vi "JGPR2.vi"() -> ()   [LabVIEW 2019]
doc: "This VI allows you to load data and graph it by raw data then gives you the fft graph and also allows for diffrent types of windowing of the data you can also look at data in frequency domain and save the data"
uses:
  <vilib>/Analysis/NI_AALPro.lvlib
panel:
  out "rate (Hz)":dbl format="%#_3g"
  in  "Window type":enum16{"Hanning", "Hamming", "Blackman"}(ring)
  out "interval (s)":dbl format="%#_3g"
  in  "Lin/dB":bool caption="Power spectrun presentation"
  in  "Tabs":T1(tab)
  out "Raw Data Graph":cluster{dbl, dbl, dbl[]}(graph)
  out "Data to FFT":cluster{dbl, dbl, "Windowed X":dbl[]}(graph)
  out "Power Spectrum":cluster{dbl, "df":dbl, "data out":dbl[]}(graph)
  out "data to save":dbl[][](array[numeric]) format="%#_3e"
  in  "Comments for header":string="This data is ....."
  in  "Windowing":bool
  out "raw data":dbl[][](array[numeric])
  out "Raw Data File Header":string
  in  "exit without save":bool
  in  "exit early":bool
  in  "save data":bool
  in  "load raw data":bool
  # "Post-processing of Data"
  # "Source data"
  # "File Output"
  # "raw"
  # "into PS"
  # "out of PS"
  # "Juan Gamez\nP3600\nCSUSB Physics"
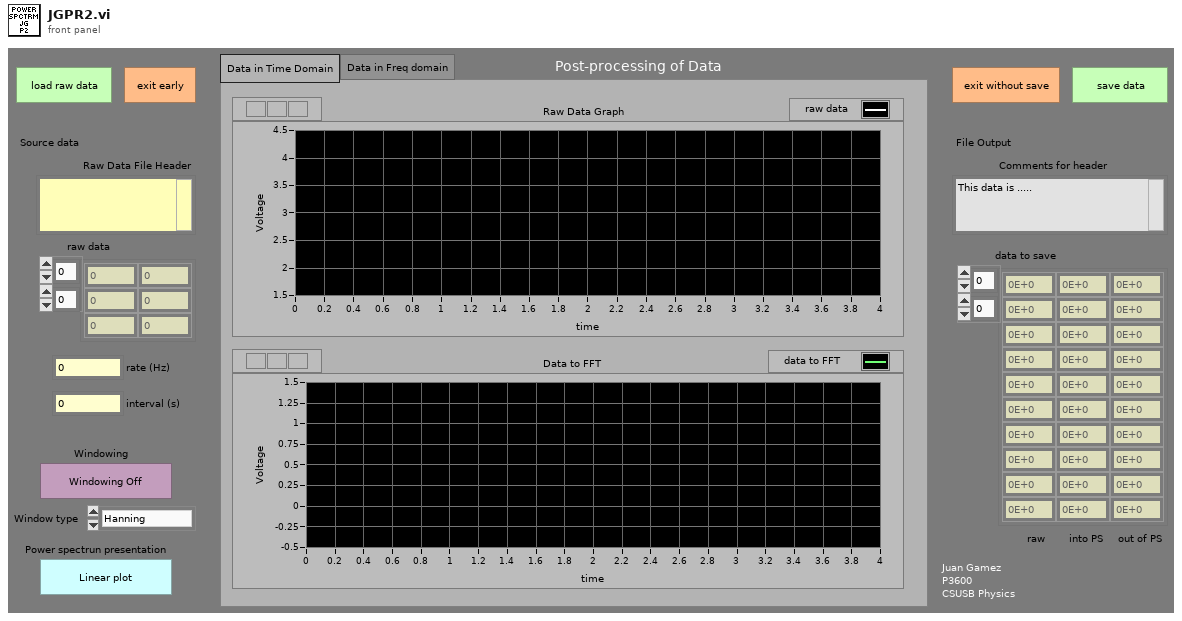
[diagram p1: front panel]
types:
  T1 = enum32{"Data in Time Domain", "Data in Freq domain"}
  T2 = cluster{dbl, "Interval (s)":dbl, "windowed data out":dbl[]}
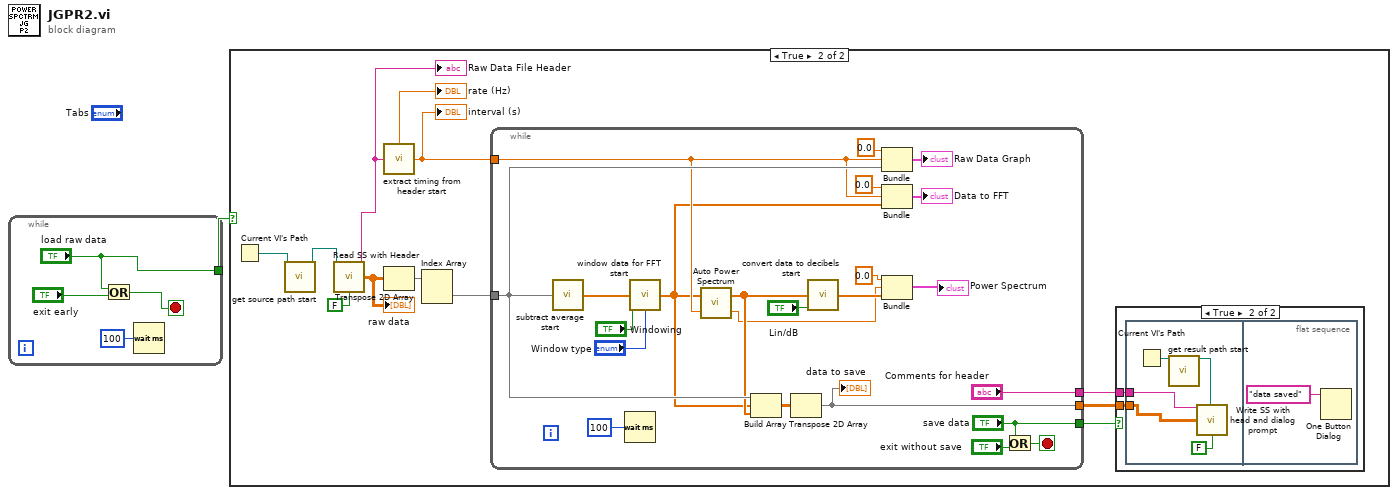
[diagram p0: block diagram]
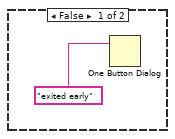
[diagram p2: hidden frame]
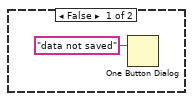
[diagram p3: hidden frame]
diagram:
  n1 = while {
    tunnel: ["load raw data"] -> w1
    stop <- w3 stop-if-true
    n2 = Or(x="load raw data", y="exit early") -> (x .or. y?=w3:bool)
    n3 = Wait (ms)(milliseconds to wait=u32 100) -> ()  [unwired: 1 out]
  }
  n4 = case shown="True" w1 {
    frame False {
      n5 = One Button Dialog(message="exited early") -> ()  [unwired: 1 in, 1 out]
    }
    frame True {
      n6 = Current VI's Path() -> (path=w11:path)
      n7 = call "get source path start.vi"("main VI path"=w11) -> ("source file path"=w10:path)  [unwired: 14 in]
      n8 = call "Read SS with Header.vi"("file path"=w10, "use int dialog (default=T)"=FALSE) -> ("Header String"=w14:string, "Data Read"=w18:dbl[][])  [unwired: 11 in, 1 out]
      "raw data" <- w18
      "Raw Data File Header" <- w14
      n9 = call "extract timing from header start.vi"("Header String"=w14) -> ("Rate (Hz)"=→"rate (Hz)":dbl, "Interval (s)"=w13:dbl)  [unwired: 13 in]
      "interval (s)" <- w13
      n10 = Transpose 2D Array(2D array=w18) -> (transposed array=w17:dbl[][])
      n11 = Index Array(array=w17) -> (element=w16:dbl[])  [unwired: 2 in]
      n12 = while {
        tunnel: w16 -> [w41]
        tunnel: ["save data"] -> w9
        tunnel: [w46] -> w7
        tunnel: ["Comments for header"] -> w8
        tunnel: w13 -> [w36]
        stop <- w48 stop-if-true
        n13 = call "subtract average start.vi"("data in"=w41) -> ("data with zero average out"=w35:dbl[])  [unwired: 14 in]
        n14 = Wait (ms)(milliseconds to wait=u32 100) -> ()  [unwired: 1 out]
        n15 = call "window data for FFT start.vi"("data in"=w35, "Windowing ON"="Windowing", "Window type"="Window type") -> ("windowed data out"=w34:dbl[])  [unwired: 12 in]
        n16 = call <vilib>:"Auto Power Spectrum.vi"("dt"=w36, "Signal (V)"=w34) -> ("df"=w29:dbl, "Power Spectrum (V^2 rms)"=w40:dbl[])
        n17 = Build Array(w41, w34, w40) -> (w39:dbl[][])
        n18 = Transpose 2D Array(2D array=w39) -> (transposed array=w46:dbl[][])
        "data to save" <- w46
        n19 = call "convert data to decibels start.vi"("data in"=w40, "Lin/dB"="Lin/dB") -> ("data out"=w30:dbl[])  [unwired: 13 in]
        n20 = Bundle(0.0, "Interval (s)"=w36, w41) -> (→"Raw Data Graph":cluster{dbl, "Interval (s)":dbl, dbl[]})  [unwired: 1 in]
        n21 = Bundle(0.0, "Interval (s)"=w36, "windowed data out"=w34) -> (→"Data to FFT":T2)  [unwired: 1 in]
        n22 = Bundle(0.0, "df"=w29, "data out"=w30) -> (→"Power Spectrum":cluster{dbl, "df":dbl, "data out":dbl[]})  [unwired: 1 in]
        n23 = Or(x="save data", y="exit without save") -> (x .or. y?=w48:bool)
      }
      n24 = case shown="True" w9 {
        tunnel: w8 -> [_ w21]
        tunnel: w7 -> [_ w20]
        frame False {
          n25 = One Button Dialog(message="data not saved") -> ()  [unwired: 1 in, 1 out]
        }
        frame True {
          n26 = flat-sequence {
            tunnel: w21 -> [w23]
            tunnel: w20 -> [w22]
            frame #0 {
              n27 = Current VI's Path() -> (path=w26:path)
              n28 = call "get result path start.vi"("main VI path"=w26) -> ("result file path"=w24:path)  [unwired: 14 in]
              n29 = call "Write SS with head and dialog prompt.vi"("Header String"=w23, "file path"=w24, "Data to Write"=w22, "use int dialog (default=T)"=FALSE) -> ()  [unwired: 12 in]
            }
            frame #1 {
              n30 = One Button Dialog(message="data saved") -> ()  [unwired: 1 in, 1 out]
            }
          }
        }
      }
    }
  }
